vi "generateEventsMeasurementsSD.vi"(0 "Measure event":refnum<user-event>, 1 "Operate":bool, 2 "Measure finished":refnum<user-event>, 3 "error in (no error)":errorcluster, 4 "Experiment in":refnum<class "Experiment.lvclass">) -> (5 "error out":errorcluster)   [LabVIEW 2015]
uses:
  Classes/Experiment.lvclass
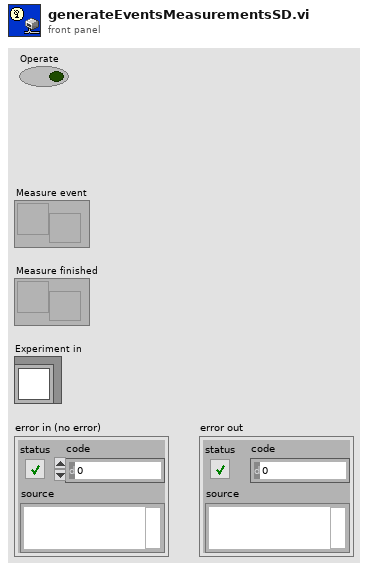
[diagram p1: front panel]
types:
  T1 = cluster{"Operate":bool, "Experiment in":refnum<class "Experiment.lvclass">}
  T2 = cluster{"Operate":bool, "Experiment in":refnum<class "Experiment.lvclass">, path}
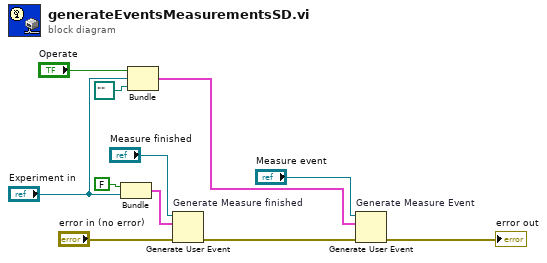
[diagram p0: block diagram]
diagram:
  n1 = Bundle("Operate"=FALSE, "Experiment in"="Experiment in") -> (w6:T1)  [unwired: 1 in]
  n2 = Bundle("Operate"="Operate", "Experiment in"="Experiment in", path "") -> (w4:T2)  [unwired: 1 in]
  n3 = Generate User Event "Generate Measure finished"(user event="Measure finished", event data cluster=w6, error in="error in (no error)") -> (error out=w11:errorcluster)  [unwired: 1 in, 1 out]
  n4 = Generate User Event "Generate Measure Event"(user event="Measure event", event data cluster=w4, error in=w11) -> (error out=→"error out":errorcluster)  [unwired: 1 in, 1 out]
